vi "keyboard_FGV.vi"(6 "Prefix":string, 7 "Action":T1, 8 "Error In":errorcluster, 9 "Unit":string, 10 "Decimal":string, 11 "Number":string) -> (0 "Error Out":errorcluster, 1 "Unit":bool, 2 "Unit msg":string, 3 "Indicator Text":string)   [LabVIEW 2021, in "Signal.lvlib"]
doc: "This FGV is used to remember the keyboard commands."
uses:
  Signal.lvlib
  Tipski Definicii/Keyboard_Sostojbi.ctl
  Tipski Definicii/check.ctl
panel:
  # "Input"
  # "Output"
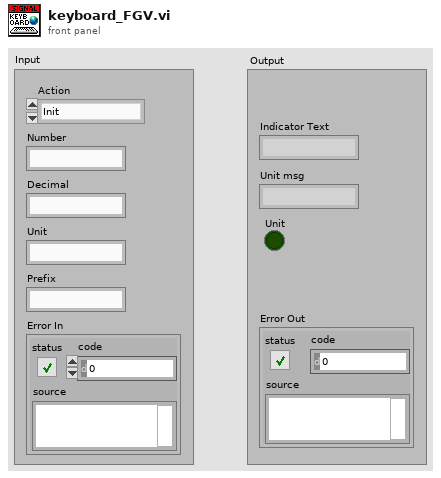
[diagram p1: front panel]
types:
  T1 = typedef "Keyboard_Sostojbi.ctl" = enum16{"Init", "Add Number", "Add Decimal", "Add Unit ", "Clear", "Read", "Enter", "CE", "Add Unit Scale", "Check Unit", "Mul", "Div"}
  T2 = typedef "check.ctl" = enum16{"Init", "Add dot", "Add +", "Add Shift", "Check", "Reset", "Reset Shift"}
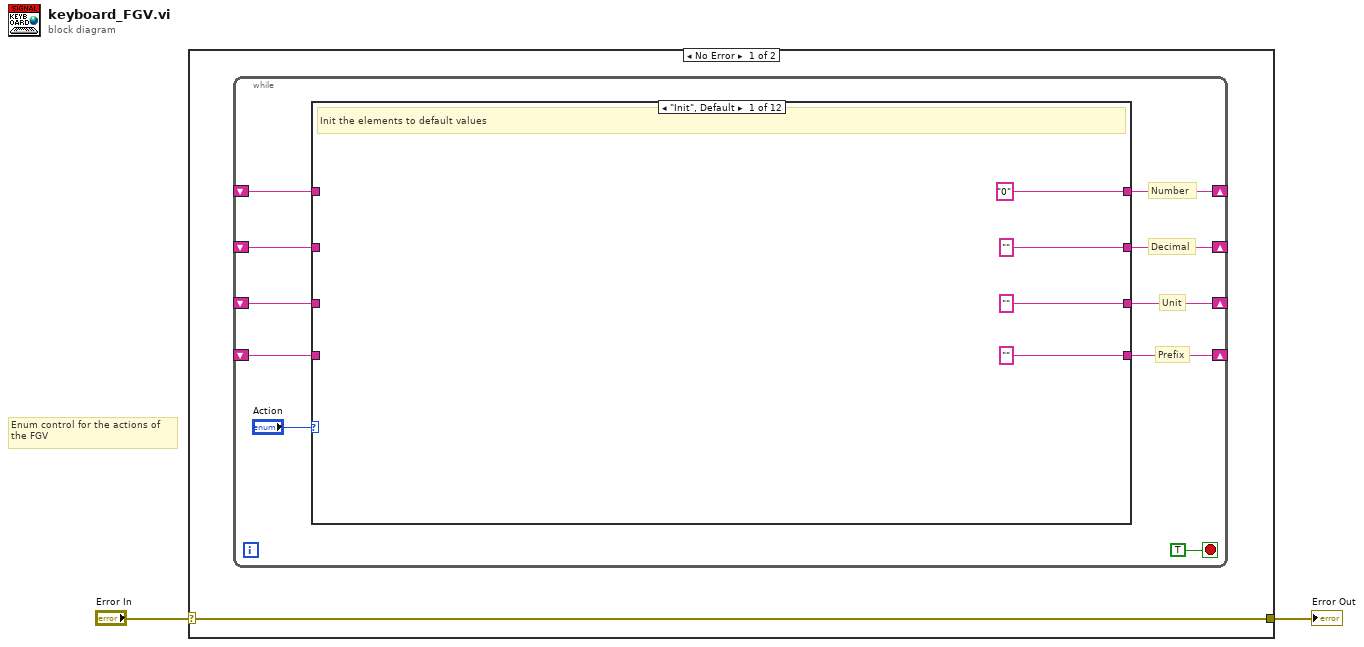
[diagram p0: block diagram]
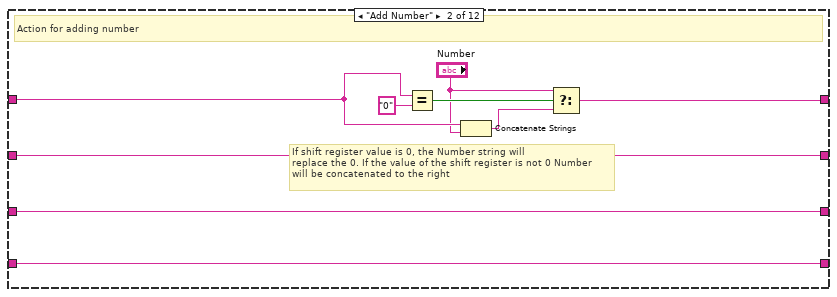
[diagram p2: hidden frame]
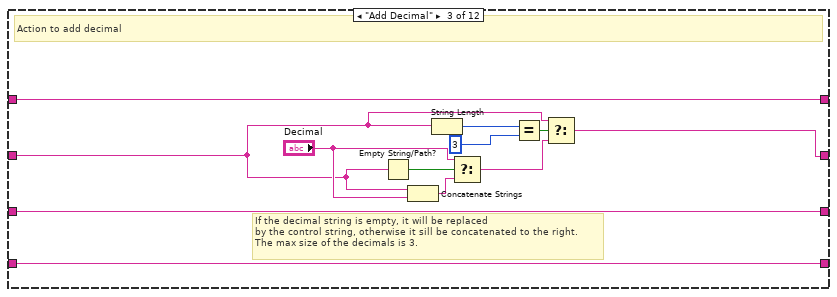
[diagram p3: hidden frame]
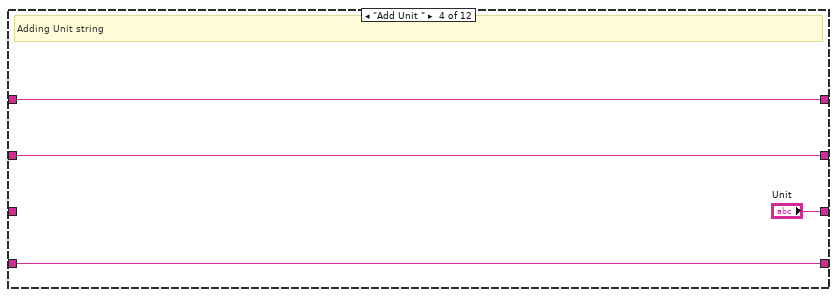
[diagram p4: hidden frame]
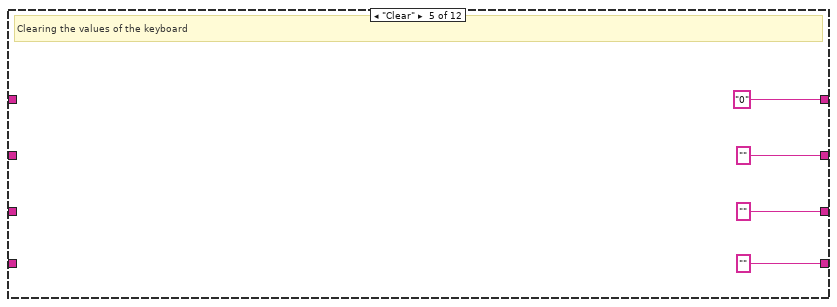
[diagram p5: hidden frame]
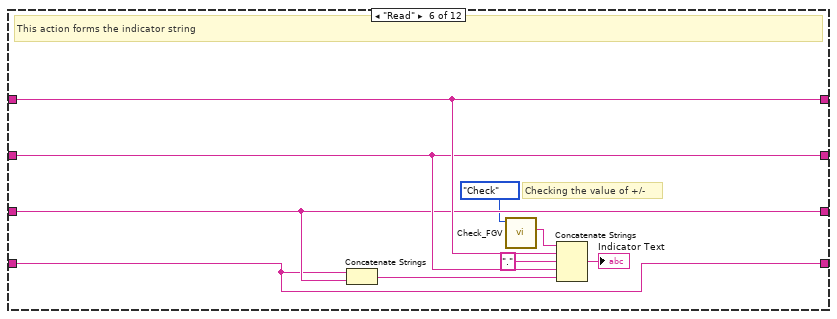
[diagram p6: hidden frame]
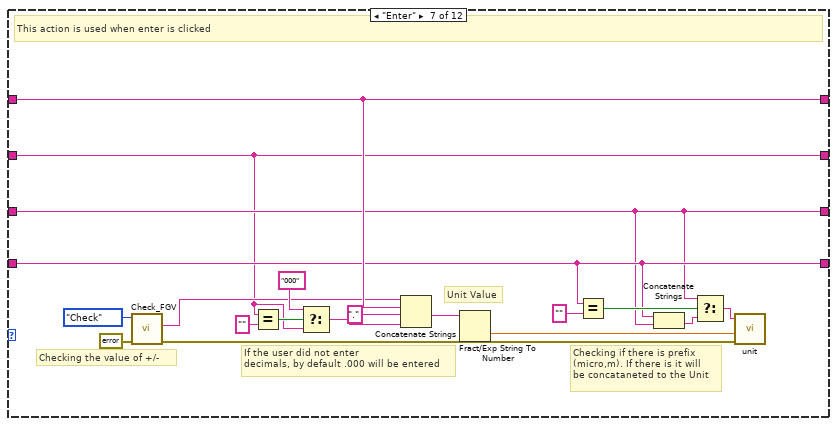
[diagram p7: hidden frame]
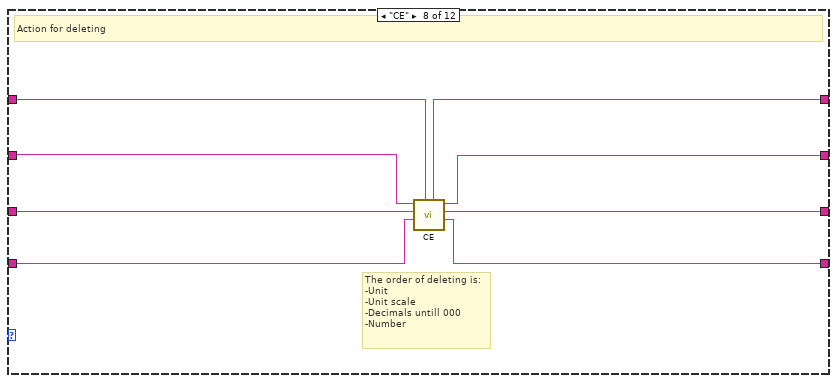
[diagram p8: hidden frame]
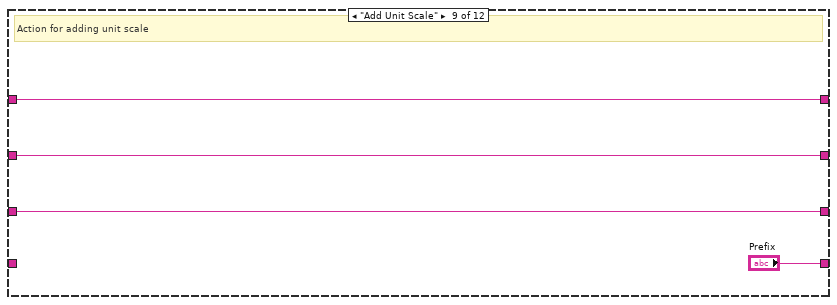
[diagram p9: hidden frame]
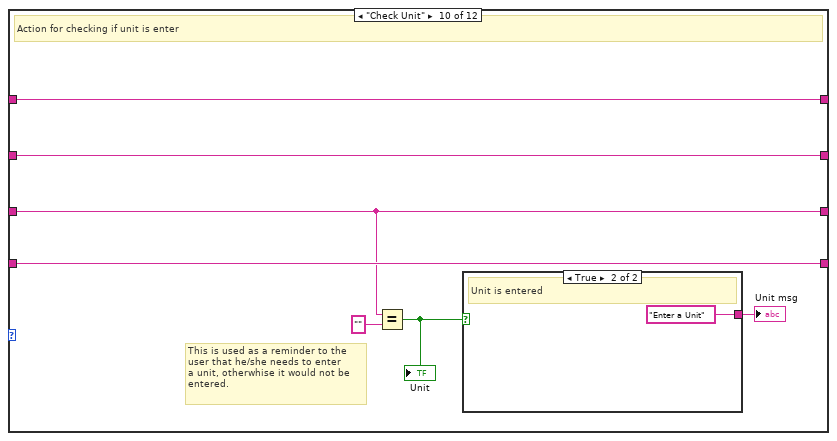
[diagram p10: hidden frame]
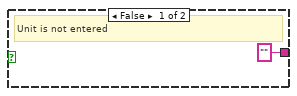
[diagram p11: hidden frame]
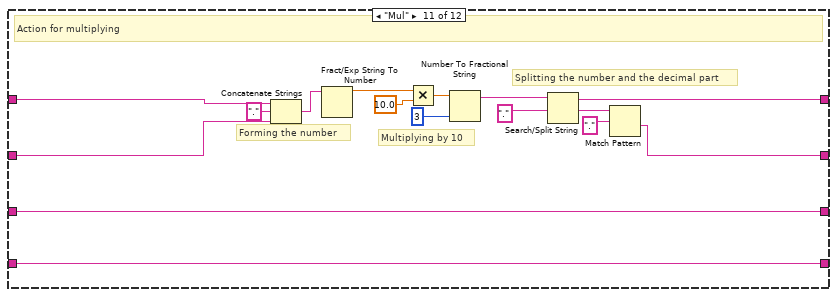
[diagram p12: hidden frame]
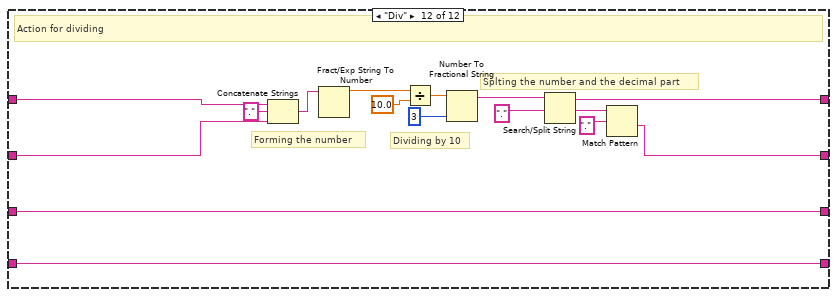
[diagram p13: hidden frame]
diagram:
  # "Enum control for the actions of\nthe FGV"
  n1 = case shown="No Error" "Error In" {
    selector: "Error In" -> [w3 w128]
    tunnel: [w3 w128] -> w1
    frame No Error {
      n2 = while {
        shift-right: [w7] -> _
        shift-left: _ -> [w10]
        shift-right: [w6] -> _
        shift-left: _ -> [w9]
        shift-right: [w12] -> _
        shift-left: _ -> [w8]
        shift-right: [w5] -> _
        shift-left: _ -> [w4]
        stop <- TRUE stop-if-true
        # "Prefix"
        # "Unit"
        # "Decimal"
        # "Number"
        n3 = case shown="\"Init\", Default" "Action" {
          tunnel: ["" w26 w29 w41 "" ("Decimal") w53 w57 w78 w84 w92 w98 w112] -> w6
          tunnel: ["" ("Unit") w25 w38 "Unit" "" ("Unit") w50 w63 w76 w85 w90 w111 w127] -> w12
          tunnel: ["0" ("Number") w19 w37 w42 "0" ("Number") w55 w74 w81 w83 w93 w97 w113] -> w7
          tunnel: w10 -> [_ w22 w37 w42 _ w55 w74 w82 w83 w93 w96 w115]
          tunnel: w9 -> [_ w26 w28 w41 _ w53 w57 w80 w84 w92 w99 w114]
          tunnel: w8 -> [_ w25 w38 _ _ w50 w63 w79 w85 w90 w111 w127]
          tunnel: ["" ("Unit") w18 w36 w39 "" ("Unit") w48 w64 w75 "Prefix" w91 w110 w126] -> w5
          tunnel: w4 -> [_ w18 w36 w39 _ w48 w64 w77 _ w91 w110 w126]
          frame "Init", Default {
            # "Init the elements to default values"
          }
          frame "Add Number" {
            # "If shift register value is 0, the Number string will\nreplace the 0. If the value of the shift register is not 0 Number\nwill be concatenated to the right"
            # "Action for adding number"
            n4 = Equal?(x=w22, y="0") -> (x = y?=w23:bool)
            n5 = Concatenate Strings(w22, "Number") -> (w20:string)
            n6 = Select(t="Number", s=w23, f=w20) -> (s? t:f=w19:string)
          }
          frame "Add Decimal" {
            # "If the decimal string is empty, it will be replaced \nby the control string, otherwise it sill be concatenated to the right.\nThe max size of the decimals is 3."
            # "Action to add decimal"
            n7 = Empty String/Path?(string/path=w28) -> (empty?=w27:bool)
            n8 = Concatenate Strings(w28, "Decimal") -> (w34:string)
            n9 = String Length(string=w28) -> (length=w33:i32)
            n10 = Select(t="Decimal", s=w27, f=w34) -> (s? t:f=w30:string)
            n11 = Equal?(x=w33, y=3) -> (x = y?=w31:bool)
            n12 = Select(t=w28, s=w31, f=w30) -> (s? t:f=w29:string)
          }
          frame "Add Unit " {
            # "Adding Unit string"
          }
          frame "Clear" {
            # "Clearing the values of the keyboard"
          }
          frame "Read" {
            # "Checking the value of +/-"
            # "This action forms the indicator string"
            n13 = Concatenate Strings(w48, w50) -> (w49:string)
            n14 = call "Check_FGV.vi"("Action"=check."Check") -> ("+- Out"=w51:string)  [unwired: 6 in, 4 out]
            n15 = Concatenate Strings(w51, w55, "." ("string"), w53, w49) -> (→"Indicator Text":string)
          }
          frame "Enter" {
            # "Unit Value"
            # "Checking if there is prefix\n(micro,m). If there is it will\nbe concataneted to the Unit"
            # "If the user did not enter \ndecimals, by default .000 will be entered"
            # "Checking the value of +/-"
            # "This action is used when enter is clicked"
            n16 = call "Check_FGV.vi"("Error In"=errorcluster {"status"=FALSE, "code"=0, "source"=""}, "Action"=check."Check") -> ("Error Out"=w69:errorcluster, "+- Out"=w59:string)  [unwired: 5 in, 3 out]
            n17 = Equal?(x=w57, y="") -> (x = y?=w61:bool)
            n18 = Select(t="000", s=w61, f=w57) -> (s? t:f=w58:string)
            n19 = Concatenate Strings(w59, w74, "." ("string"), w58) -> (w72:string)
            n20 = Fract/Exp String To Number(string=w72) -> (number=w71:dbl)  [unwired: 3 in, 1 out]
            n21 = Equal?(x=w64, y="") -> (x = y?=w67:bool)
            n22 = Concatenate Strings(w64, w63) -> (w65:string)
            n23 = Select(t=w63, s=w67, f=w65) -> (s? t:f=w66:string)
            n24 = call "unit.vi"("Error In"=w69, "Signal Amp"=w71, "Unit"=w66) -> ()  [unwired: 8 in, 1 out]
          }
          frame "CE" {
            # "The order of deleting is:\n-Unit\n-Unit scale\n-Decimals untill 000\n-Number"
            # "Action for deleting"
            n25 = call "CE.vi"("Number in"=w82, "Unit scale In"=w77, "Unit in"=w79, "Decimal in"=w80) -> ("Unit scale out"=w75:string, "Unit out"=w76:string, "Decimal out"=w78:string, "Number out"=w81:string)  [unwired: 3 in, 1 out]
          }
          frame "Add Unit Scale" {
            # "Action for adding unit scale"
          }
          frame "Check Unit" {
            # "This is used as a reminder to the\nuser that he/she needs to enter \na unit, otherwhise it would not be\nentered."
            # "Action for checking if unit is enter"
            n26 = Equal?(x=w90, y="") -> (x = y?=w88:bool)
            "Unit" <- w88
            n27 = case shown="True" w88 {
              tunnel: ["" "Enter a Unit"] -> w87
              frame False {
                # "Unit is not entered"
              }
              frame True {
                # "Unit is entered"
              }
            }
            "Unit msg" <- w87
          }
          frame "Mul" {
            # "Splitting the number and the decimal part"
            # "Multiplying by 10"
            # "Forming the number"
            # "Action for multiplying"
            n28 = Concatenate Strings(w96, "." ("string"), w99) -> (w108:string)
            n29 = Fract/Exp String To Number(string=w108) -> (number=w107:dbl)  [unwired: 3 in, 1 out]
            n30 = Multiply(x=w107, y=10.0) -> (x*y=w105:dbl)
            n31 = Number To Fractional String(number=w105, precision (6)=i16 3) -> (F-format string=w103:string)  [unwired: 2 in]
            n32 = Search/Split String(string=w103, search string/char (-)="." ("regular expression")) -> (substring before match=w97:string, match + rest of string=w100:string)  [unwired: 1 in, 1 out]
            n33 = Match Pattern(string=w100, regular expression=".") -> (after substring=w98:string)  [unwired: 1 in, 3 out]
          }
          frame "Div" {
            # "Splting the number and the decimal part"
            # "Dividing by 10"
            # "Forming the number"
            # "Action for dividing"
            n34 = Concatenate Strings(w115, "." ("string"), w114) -> (w124:string)
            n35 = Fract/Exp String To Number(string=w124) -> (number=w123:dbl)  [unwired: 3 in, 1 out]
            n36 = Divide(x=w123, y=10.0) -> (x/y=w121:dbl)
            n37 = Number To Fractional String(number=w121, precision (6)=i16 3) -> (F-format string=w119:string)  [unwired: 2 in]
            n38 = Search/Split String(string=w119, search string/char (-)="." ("regular expression")) -> (substring before match=w113:string, match + rest of string=w116:string)  [unwired: 1 in, 1 out]
            n39 = Match Pattern(string=w116, regular expression=".") -> (after substring=w112:string)  [unwired: 1 in, 3 out]
          }
        }
      }
    }
    frame Error {
    }
  }
  "Error Out" <- w1
